vi "Modify.vi"(6 "Max Lines Per File":i32, 8 "error in (no error)":errorcluster, 10 "Directory":path, 11 "Log in":refnum<class "Log.lvclass">) -> (0 "error out":errorcluster, 3 "Log out":refnum<class "Log.lvclass">)   [LabVIEW 2020, in "Log.lvclass"]
doc: "Sets up the class to beging logging.\n\nThe input file path is checked and all the necessary directories in the chain are created.\n\nThis VI also writes the header to the file."
uses:
  Log.lvclass
  Log.lvclass/Log.ctl
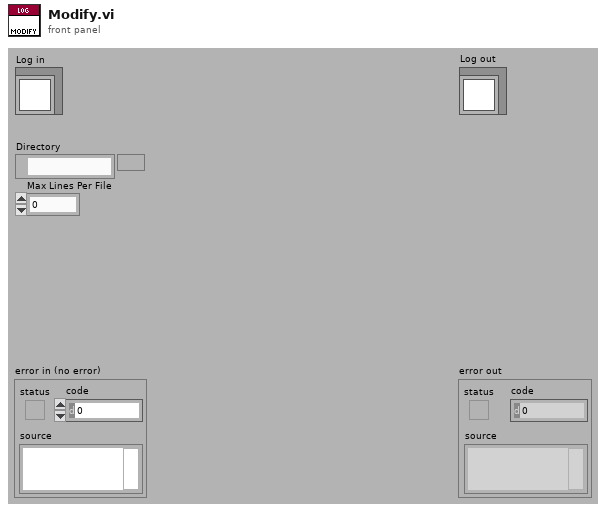
[diagram p1: front panel]
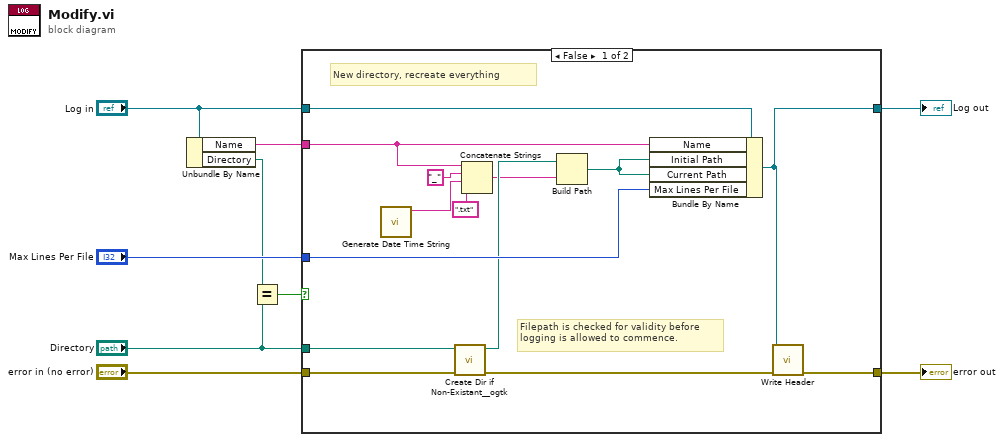
[diagram p0: block diagram]
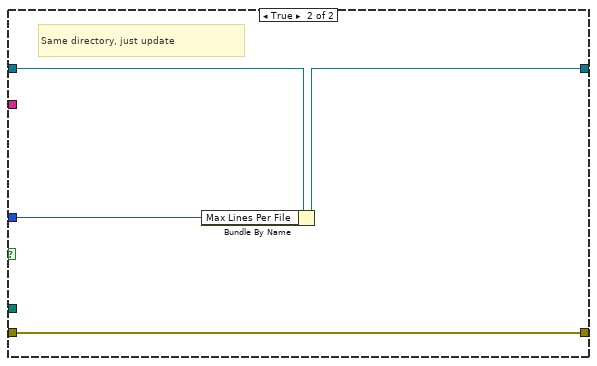
[diagram p2: hidden frame]
diagram:
  n1 = Unbundle By Name("Log in") -> ("Name"=w1:string, "Directory"=w3:path)
  n2 = Equal?(x=w3, y="Directory") -> (x = y?=w2:bool)
  n3 = case shown="False" w2 {
    tunnel: "error in (no error)" -> [w23 w24]
    tunnel: "Max Lines Per File" -> [w22 w25]
    tunnel: [w20 w24] -> w8
    tunnel: [w10 w26] -> w7
    tunnel: "Log in" -> [w13 w27]
    tunnel: "Directory" -> [w12 _]
    tunnel: w1 -> [w11 _]
    frame False {
      # "New directory, recreate everything"
      # "Filepath is checked for validity before logging is allowed to commence."
      n4 = call "Generate Date Time String.vi"() -> ("Date time string"=w14:string)  [unwired: 10 in, 1 out]
      n5 = call <userlib>:"Create Dir if Non-Existant__ogtk.vi"("error in (no error)"=w23, "Directory Path"=w12) -> ("error out"=w21:errorcluster, "dup Directory Path"=w18:path)  [unwired: 1 in, 7 out]
      n6 = Concatenate Strings(w11, "_" ("string"), w14, ".txt" ("string")) -> (w17:string)
      n7 = Build Path(base path=w18, name or relative path=w17) -> (appended path=w16:path)
      n8 = Bundle By Name(cluster=w13, "Name"=w11, "Initial Path"=w16, "Current Path"=w16, "Max Lines Per File"=w22) -> (w10:refnum<class "Log.lvclass">)
      n9 = call "Write Header.vi"("error in (no error)"=w21, "Log in"=w10) -> ("error out"=w20:errorcluster)  [unwired: 1 in, 8 out]
    }
    frame True {
      # "Same directory, just update"
      n10 = Bundle By Name(cluster=w27, "Max Lines Per File"=w25) -> (w26:refnum<class "Log.lvclass">)
    }
  }
  "error out" <- w8
  "Log out" <- w7
